vi "外观.vi"(0 "Data In":T4 caption="数据输入", 2 "Display State In":T2 caption="显示状态输入", 3 "Container State":T3 caption="容器状态") -> (6 "Data Out":T4 caption="数据输出", 7 "Display State Out":T2 caption="显示状态输出", 8 "Action":T1 caption="动作")   [LabVIEW 2016, in "自定义多列表框.xctl"]
uses:
  <vilib>/_xctls/Container State.ctl
  <vilib>/_xctls/Action.ctl
  listbox/listbox.lvclass
  LNK/Copy/Copy.lvclass
  LNK/Delete/Delete.lvclass
  LNK/UP/UP.lvclass
  LNK/Down/Down.lvclass
  LNK/Show Row/Show Row.lvclass
  LNK/Hide Row/Hide Row.lvclass
  LNK/Parent Class/Menu.lvclass
  listbox/listbox.lvclass/listbox.ctl
  <vilib>/_xctls/XControlSupport.lvlib
panel:
  in  "多列列表框":i32(listbox)
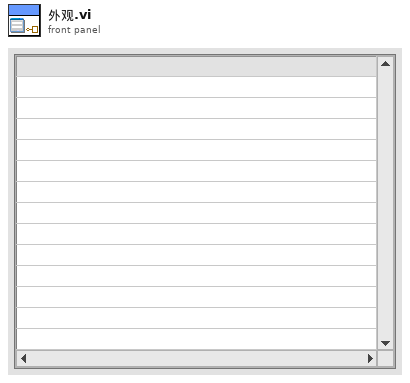
[diagram p1: front panel]
types:
  T1 = typedef "XControlSupport.lvlib/Action.ctl" = cluster{"Data Changed?":bool, "State Changed?":bool, "Action Name":string}
  T2 = typedef "自定义多列表框.xctl/状态.ctl" = cluster{"数组":string[][]}
  T3 = typedef "XControlSupport.lvlib/Container State.ctl" = cluster{"Indicator?":bool, "Run Mode?":bool, " Refnum":refnum<vi>}
  T4 = typedef "自定义多列表框.xctl/数据.ctl" = cluster{"行首":string[], "列首":string[], "项名":string[][]}
  T5 = typedef "LVPoint32TypeDef.ctl" = cluster{"Horizontal":i32, "Vertical":i32}
  T6 = typedef "LVRowAndColumnTypeDef.ctl" = cluster{"Row":i32, "Column":i32}
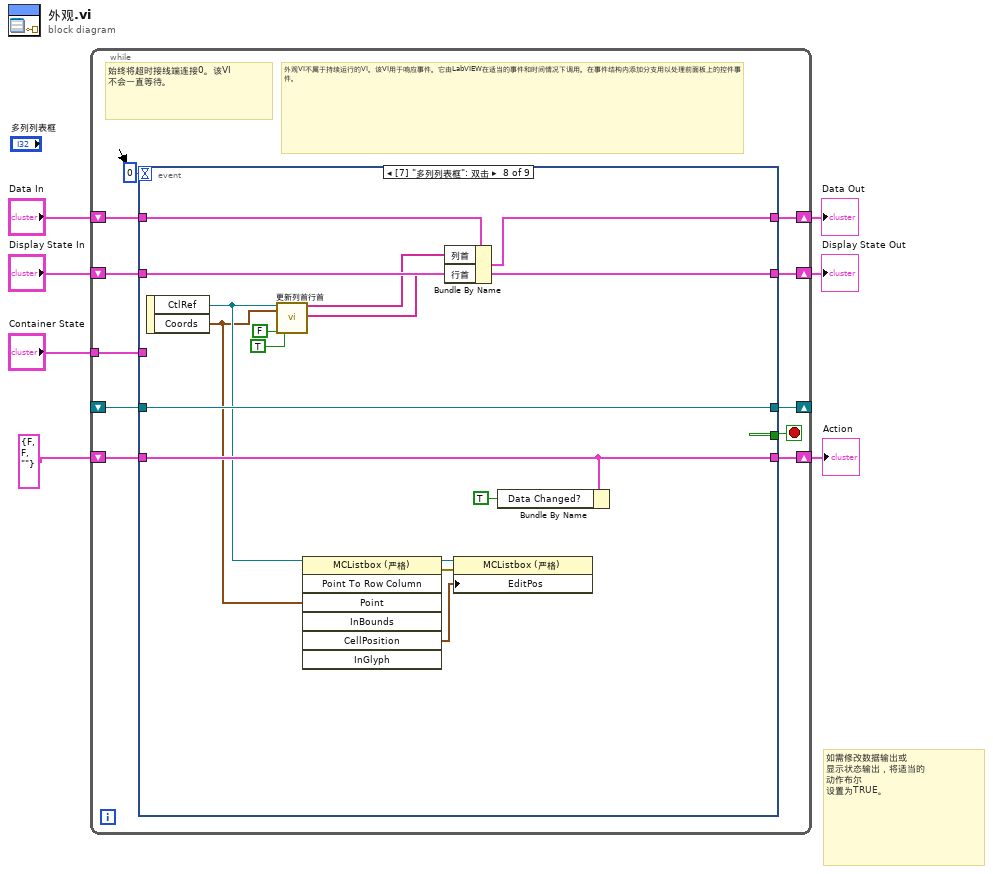
[diagram p0: block diagram]
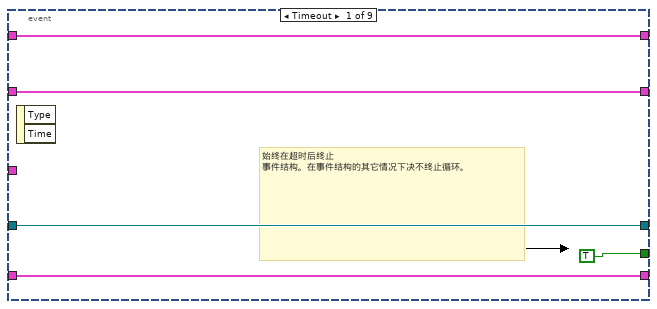
[diagram p2: hidden frame]
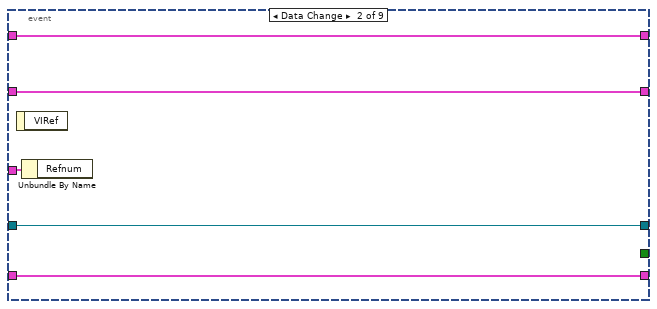
[diagram p3: hidden frame]
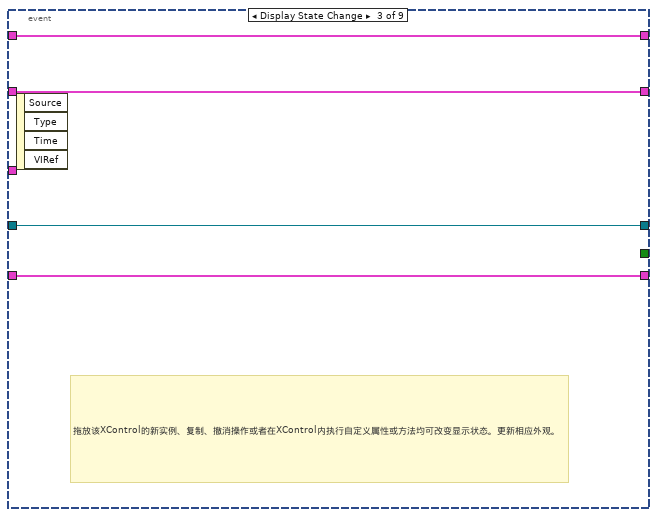
[diagram p4: hidden frame]
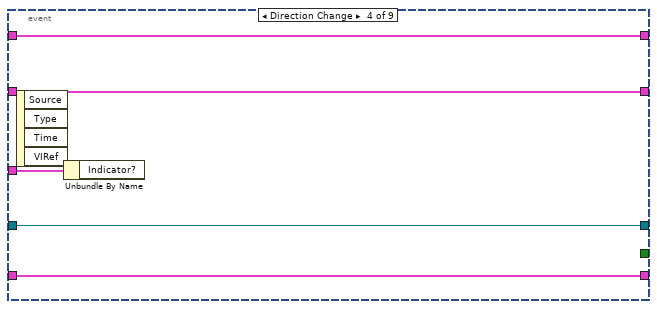
[diagram p5: hidden frame]
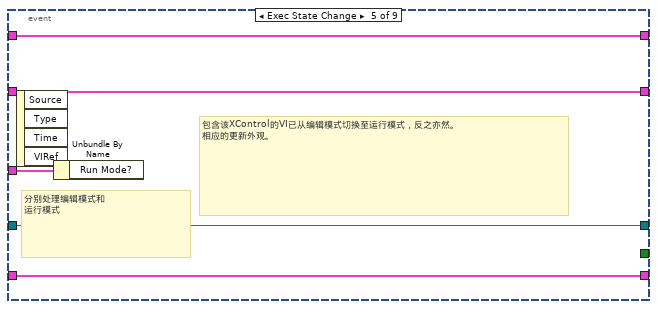
[diagram p6: hidden frame]
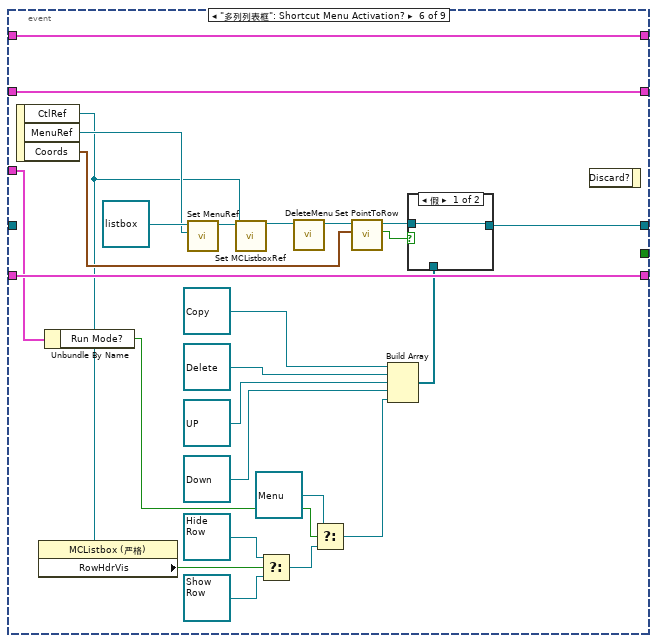
[diagram p7: hidden frame]
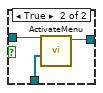
[diagram p8: hidden frame]
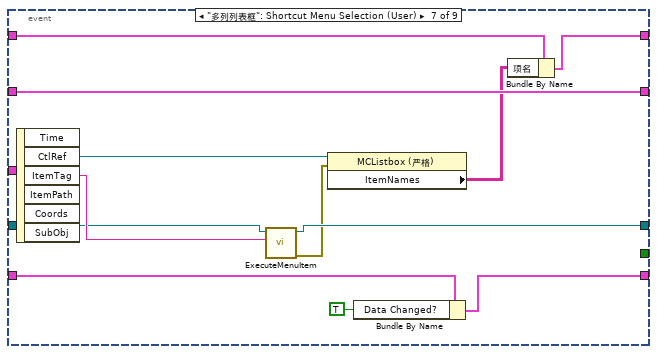
[diagram p9: hidden frame]
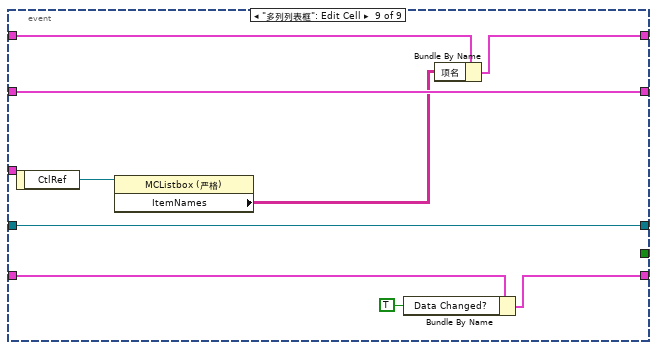
[diagram p10: hidden frame]
diagram:
  # "如需修改数据输出或\n显示状态输出，将适当的\n动作布尔\n设置为TRUE。"
  n1 = while {
    shift-right: [w17] -> w4
    shift-left: "Display State In" -> [w18]
    tunnel: "Container State" -> [w14]
    shift-right: [w12] -> w7
    shift-left: "Data In" -> [w13]
    shift-right: [w10] -> w2
    shift-left: T1 {"Data Changed?"=FALSE, "State Changed?"=FALSE, "Action Name"=""} ("Action") -> [w11]
    shift-right: [w9] -> _
    shift-left: _ -> [w8]
    stop <- w16 stop-if-true
    # "外观VI不属于持续运行的VI。该VI用于响应事件。它由LabVIEW在适当的事件和时间情况下调用。在事件结构内添加分支用以处理前面板上的控件事件。"
    # "始终将超时接线端连接0。该VI\n不会一直等待。"
    n2 = event shown="[7] \"多列列表框\": 双击" {
      selector: _ -> [_ _ _ _ _ _ _ _ _]
      dyn-events: _ -> [_ _ _ _ _ _ _ _ _]
      timeout: 0 -> [_ _ _ _ _ _ _ _ _]
      tunnel: w18 -> [w21 w28 w32 w36 w41 w68 w84 w99 w103]
      tunnel: [w21 w28 w32 w36 w41 w68 w84 w99 w103] -> w17
      tunnel: [TRUE _ _ _ _ _ _ _ _] -> w16
      tunnel: w14 -> [_ w25 _ w37 w42 w50 _ _ _]
      tunnel: w13 -> [w20 w24 w29 w33 w40 w67 w75 w96 w101]
      tunnel: [w20 w24 w29 w33 w40 w67 w74 w95 w100] -> w12
      tunnel: [w22 w27 w31 w35 w39 w66 w78 w92 w105] -> w10
      tunnel: w11 -> [w22 w27 w31 w35 w39 w66 w79 w92 w106]
      tunnel: [w19 w26 w30 w34 w38 w52 w81 w98 w104] -> w9
      tunnel: w8 -> [w19 w26 w30 w34 w38 _ w82 w98 w104]
      event Timeout {
        # "始终在超时后终止\n事件结构。在事件结构的其它情况下决不终止循环。"
        n3 = event-data() -> ()  [unwired: 1 in, 2 out]
      }
      event Data Change {
        n4 = event-data() -> ()  [unwired: 1 in, 1 out]
        n5 = Unbundle By Name(w25) -> ()  [unwired: 1 out]
      }
      event Display State Change {
        # "拖放该XControl的新实例、复制、撤消操作或者在XControl内执行自定义属性或方法均可改变显示状态。更新相应外观。"
        n6 = event-data() -> ()  [unwired: 1 in, 4 out]
      }
      event Direction Change {
        n7 = event-data() -> ()  [unwired: 1 in, 4 out]
        n8 = Unbundle By Name(w37) -> ()  [unwired: 1 out]
      }
      event Exec State Change {
        # "包含该XControl的VI已从编辑模式切换至运行模式，反之亦然。\n相应的更新外观。"
        # "分别处理编辑模式和\n运行模式"
        n9 = event-data() -> ()  [unwired: 1 in, 4 out]
        n10 = Unbundle By Name(w42) -> ()  [unwired: 1 out]
      }
      event "多列列表框": Shortcut Menu Activation? {
        n11 = event-data() -> ("CtlRef"=w51:refnum<vi>, "MenuRef"=w63:refnum<k9>, "Coords"=w55:T5)  [unwired: 1 in]
        n12 = property class="MCListbox (严格)"(reference=w51) -> ("RowHdrVis"=w49:bool)  [unwired: 1 in, 2 out]
        n13 = Unbundle By Name(w50) -> ("Run Mode?"=w46:bool)
        n14 = call "Set MenuRef.vi"("MenuRef"=w63, "listbox in"=refnum<class "listbox.lvclass"> refnum ("listbox.lvclass")) -> ("listbox out"=w64:refnum<class "listbox.lvclass">)  [unwired: 9 in]
        n15 = call "Set MCListboxRef.vi"("MCListboxRef"=w51, "listbox in"=w64) -> ("listbox out"=w62:refnum<class "listbox.lvclass">)  [unwired: 9 in]
        n16 = Select(t=refnum<class "Hide Row.lvclass"> refnum ("Hide Row.lvclass"), s=w49, f=refnum<class "Show Row.lvclass"> refnum ("Show Row.lvclass")) -> (s? t:f=w45:refnum<class "Menu.lvclass">)
        n17 = call "DeleteMenu.vi"("listbox 输入"=w62) -> ("listbox 输出"=w56:refnum<class "listbox.lvclass">)  [unwired: 9 in, 1 out]
        n18 = Select(t=refnum<class "Menu.lvclass"> refnum ("Menu.lvclass"), s=w46, f=w45) -> (s? t:f=w43:refnum<class "Menu.lvclass">)
        n19 = call "Set PointToRow.vi"("坐标"=w55, "listbox 输入"=w56) -> ("边界内？"=w53:bool, "listbox 输出"=w54:refnum<class "listbox.lvclass">)  [unwired: 7 in, 1 out]
        n20 = Build Array(refnum<class "Copy.lvclass"> refnum ("Copy.lvclass"), refnum<class "Delete.lvclass"> refnum ("Delete.lvclass"), refnum<class "UP.lvclass"> refnum ("UP.lvclass"), refnum<class "Down.lvclass"> refnum ("Down.lvclass"), w43) -> (w57:refnum<class "Menu.lvclass">[])
        n21 = case shown="假" w53 {
          tunnel: w57 -> [_ w72]
          tunnel: w54 -> [w69 w71]
          tunnel: [w69 w70] -> w52
          frame False {
          }
          frame True {
            n22 = call "ActivateMenu.vi"("MenuClassArray"=w72, "listbox 输入"=w71) -> ("listbox 输出"=w70:refnum<class "listbox.lvclass">)  [unwired: 8 in, 1 out]
          }
        }
        n23 = event-data() -> ()  [unwired: 2 in, 1 out]
      }
      event "多列列表框": Shortcut Menu Selection (User) {
        n24 = event-data() -> ("CtlRef"=w76:refnum<vi>, "ItemTag"=w83:string)  [unwired: 1 in, 4 out]
        n25 = call "ExecuteMenuItem.vi"("项标识符"=w83, "listbox 输入"=w82) -> ("error out"=w77:errorcluster, "listbox 输出"=w81:refnum<class "listbox.lvclass">)  [unwired: 8 in]
        n26 = property class="MCListbox (严格)"(reference=w76, error in=w77) -> ("ItemNames"=w73:string[][])  [unwired: 2 out]
        n27 = Bundle By Name(cluster=w79, "Data Changed?"=TRUE) -> (w78:T1)
        n28 = Bundle By Name(cluster=w75, "项名"=w73) -> (w74:T4)
      }
      event "多列列表框": Double Click {
        n29 = event-data() -> ("CtlRef"=w88:refnum<vi>, "Coords"=w86:T5)  [unwired: 1 in]
        n30 = call "更新列首行首.vi"("MulticolumnListbox输入"=w88, "Coords"=w86, "项名？"=FALSE, "编辑单元格"=TRUE) -> ("列首"=w94:string[], "行首"=w93:string[])  [unwired: 11 in, 3 out]
        n31 = invoke class="MCListbox (严格)" method="Point To Row Column"(reference=w88, "Point"=w86) -> (reference out=w91:refnum<vi>, error out=w90:errorcluster, "CellPosition"=w87:T6)  [unwired: 5 in, 4 out]
        n32 = Bundle By Name(cluster=w96, "列首"=w94, "行首"=w93) -> (w95:T4)
        n33 = property class="MCListbox (严格)"(reference=w91, error in=w90, "EditPos"=w87) -> ()  [unwired: 2 out]
        n34 = Bundle By Name(cluster=w92, "Data Changed?"=TRUE) -> ()  [unwired: 1 out]
      }
      event "多列列表框": Edit Cell {
        n35 = event-data() -> ("CtlRef"=w108:refnum<vi>)  [unwired: 1 in]
        n36 = property class="MCListbox (严格)"(reference=w108) -> ("ItemNames"=w102:string[][])  [unwired: 1 in, 2 out]
        n37 = Bundle By Name(cluster=w106, "Data Changed?"=TRUE) -> (w105:T1)
        n38 = Bundle By Name(cluster=w101, "项名"=w102) -> (w100:T4)
      }
    }
  }
  "Display State Out" <- w4
  "Data Out" <- w7
  "Action" <- w2
